vi "LinxI2cClose.vi"(8 "Error In":errorcluster, 10 "I2C Channel":u8, 11 "LINX Resource":T1) -> (0 "Error Out":errorcluster, 3 "LINX Resource":T1)   [LabVIEW 2014, in "LMH-LINX.lvlib" / "Local IO.lvlib"]
uses:
  Local IO.lvlib
  Type Defs/LINX Ref.ctl
  Type Defs/Platform.ctl
  Type Defs/Interface.ctl
  Device/Type Defs/LINX Device Config.ctl
  Device/Type Defs/TCP Config.ctl
  Device/Type Defs/Channels.ctl
  <vilib>/MakerHub/LINX/Private/Type Defs/Channel FGV States.ctl
  <vilib>/myRIO/Instrument Drivers/Onboard IO/I2C/typedefs/I2C Transfer Rate.ctl
  <vilib>/myRIO/Instrument Drivers/Onboard IO/I2C/I2C.lvlib
  <vilib>/myRIO/Instrument Drivers/Onboard IO/I2C/typedefs/I2C Configuration.ctl
  <vilib>/myRIO/Common/Instrument Driver Framework/myRIO v1.0/I2C/typedefs/I2C Channels Enum.ctl
  <vilib>/myRIO/Common/Instrument Driver Framework/Utilities/typedefs/Generic FPGA Reference.ctl
  <vilib>/myRIO/Common/Instrument Driver Framework/Utilities/typedefs/myRIO v1.0 Reference.ctl
  <vilib>/myRIO/Common/Instrument Driver Framework/Utilities/typedefs/Hardware Version Enum.ctl
  <vilib>/myRIO/Common/Instrument Driver Framework/Utilities/typedefs/myRIO Generic Hardware Reference.ctl
  <vilib>/myRIO/Instrument Drivers/Onboard IO/I2C/typedefs/I2C Reference.ctl
  liblinxdevice.dll
  LMH-LINX.lvlib
  Device/Device.lvlib
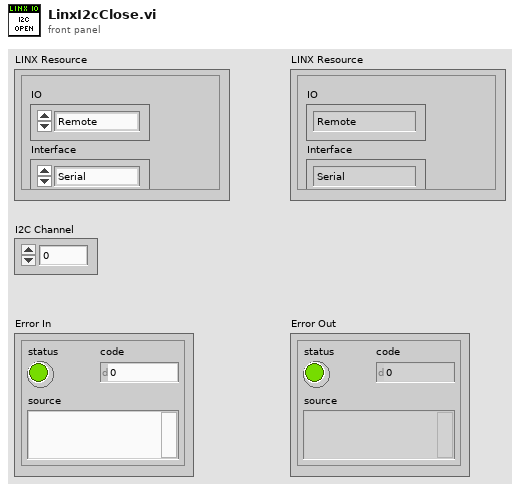
[diagram p1: front panel]
types:
  T1 = typedef "LMH-LINX.lvlib/LINX Ref.ctl" = cluster{"IO":T2, "Interface":T3, "LINX Device Config":T4}
  T2 = typedef "LMH-LINX.lvlib/Platform.ctl" = enum16{"Remote", "Local"}
  T3 = typedef "LMH-LINX.lvlib/Interface.ctl" = enum16{"Serial", "TCP"}
  T4 = typedef "LMH-LINX.lvlib/Device.lvlib/LINX Device Config.ctl" = cluster{"Interface":T3, "COM Port":refnum<visa-resource-name>, "TCP Configuration":T5, "Device Family":u8, "Device ID":u8, "Device Name":string, "TCP Ref":refnum<k5>, "Channels":T6}
  T5 = typedef "LMH-LINX.lvlib/Device.lvlib/TCP Config.ctl" = cluster{"IP Address":string, "Port":u16}
  T6 = typedef "LMH-LINX.lvlib/Channels.ctl" = cluster{"DI":u8[], "DO":u8[], "AI":u8[], "AO":u8[], "PWM":u8[], "QE":u8[], "UART":u8[], "I2C 2":u8[], "SPI":u8[], "CAN":u8[], "Servo":u8[], "AI Ref (V)":dbl, "AI Resolution (Bits)":u8, "AO Ref (V)":dbl, "AO Resolution (Bits)":u8}
  T7 = typedef "I2C.lvlib/I2C Reference.ctl" = cluster{"myRIO Reference":T8, "I2C Channels Enum":T12, "I2C Configuration":T13}
  T8 = typedef "myRIO Generic Hardware Reference.ctl" = cluster{"myRIO Model":T9, "myRIO Hardware Reference":T10}
  T9 = typedef "Hardware Version Enum.ctl" = enum16{"Unknown", "myRIO-1900", "myRIO-1950"}
  T10 = typedef "myRIO v1.0 Reference.ctl" = cluster{"Generic FPGA Reference":T11, "Allow multiple opens":bool}
  T11 = typedef "Generic FPGA Reference.ctl" = refnum<k20>
  T12 = typedef "I2C Channels Enum.ctl" = enum16{"Not Connected", "A/I2C", "B/I2C"}
  T13 = typedef "I2C.lvlib/I2C Configuration.ctl" = cluster{"I2C Transfer Rate":T14}
  T14 = typedef "I2C.lvlib/I2C Transfer Rate.ctl" = enum16{"Standard mode (100 kbps)", "Fast mode (400 kbps)"}
  T15 = typedef "LMH-LINX.lvlib/Channel FGV States.ctl" = enum16{"Initialize", "Get", "Set"}
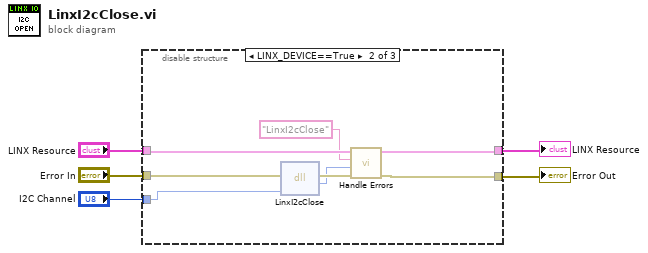
[diagram p0: block diagram]
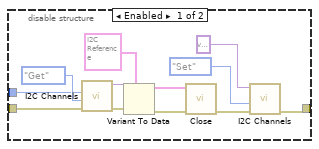
[diagram p4: hidden frame]
diagram:
  n1 = disable-structure shown="LINX_DEVICE==True" {
    disable-tunnel: "LINX Resource" -> [w7 w14 w18]
    disable-tunnel: "Error In" -> [w6 w15 w16]
    disable-tunnel: [w6 w12 w19] -> w3
    disable-tunnel: [w7 w13 w18] -> w2
    disable-tunnel: "I2C Channel" -> [_ w8 w17]
    frame condition #0 (active) {
    }
    frame condition #1 {
      n2 = dll-call lib="liblinxdevice.*" fn="LinxI2cClose"(error in=w15, "channel"=w8) -> (error out=w11:errorcluster, "LinxStatus"=w10:i32)  [unwired: 3 in, 1 out]
      n3 = call <vilib>:"Handle Errors.vi"("Error In"=w11, "LinxStatus"=w10, "Function Name"="LinxI2cClose", "LINX Resource"=w14) -> ("Error Out"=w12:errorcluster, "LINX Resource"=w13:T1)  [unwired: 6 in]
    }
    frame condition #2 {
      n4 = disable-structure shown="Disabled" {
        disable-tunnel: w16 -> [w21 w32]
        disable-tunnel: [w22 w32] -> w19
        disable-tunnel: w17 -> [w20 _]
        frame Enabled {
          n5 = call <vilib>:"I2C Channels.vi"("Error In"=w21, "Channel State"=Channel_FGV_States."Get", "Channel Number"=w20) -> ("Error Out"=w26:errorcluster, "I2C Channel"=w25:variant)  [unwired: 7 in]
          n6 = Variant To Data(error in=w26, type=T7 {"myRIO Reference"={"myRIO Model"=enum."Unknown", "myRIO Hardware Reference"={"Generic FPGA Reference"=refnum, "Allow multiple opens"=FALSE}}, "I2C Channels Enum"=enum."Not Connected", "I2C Configuration"={"I2C Transfer Rate"=enum."Standard mode (100 kbps)"}}, Variant=w25) -> (data=w30:T7, error out=w31:errorcluster)
          n7 = call <vilib>:"Close.vi"("error in (no error)"=w31, "I2C Ref In"=w30) -> ("error out"=w27:errorcluster)  [unwired: 9 in]
          n8 = call <vilib>:"I2C Channels.vi"("Error In"=w27, "Channel State"=Channel_FGV_States."Set", "I2C Channel"=variant) -> ("Error Out"=w22:errorcluster)  [unwired: 7 in, 1 out]
        }
        frame Disabled {
          # "myRIO Support Disabled"
        }
      }
    }
  }
  "Error Out" <- w3
  "LINX Resource" <- w2
